vi "FTW-MessagePayload-Serialize.vi"(0 "Message In":T1, 11 "error in":errorcluster) -> (4 "Serialized Message":string, 15 "error out":errorcluster)   [LabVIEW 2013]
uses:
  FTW-MessagePayload.ctl
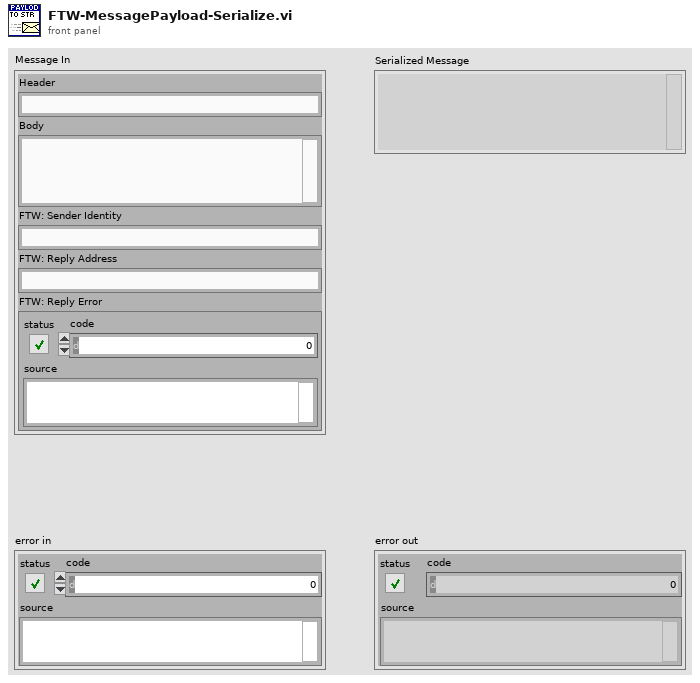
[diagram p1: front panel]
types:
  T1 = typedef "FTW-MessagePayload.ctl" = cluster{"Header":string, "Body":string, "FTW: Sender Identity":string, "FTW: Reply Address":string, "FTW: Reply Error":errorcluster}
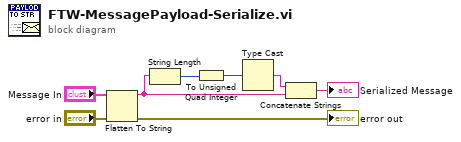
[diagram p0: block diagram]
diagram:
  n1 = Flatten To String(anything="Message In", error in (no error)="error in") -> (data string=w6:string, error out=→"error out":errorcluster)  [unwired: 2 in, 1 out]
  n2 = String Length(string=w6) -> (length=w8:i32)
  n3 = To Unsigned Quad Integer(1:w8) -> (0:w5:u64)
  n4 = Type Cast(x=w5) -> (*(type *) &x=w7:string)  [unwired: 1 in]
  n5 = Concatenate Strings(w7, w6) -> (→"Serialized Message":string)
